vi "StageController.vi"() -> ()   [LabVIEW 2013]
panel:
  in  "Motor Port":i32=14 min=1 max=255 step=1
  out "Port\nOpen\nStatus 2":bool
  in  "moveForward":bool caption="Move Forward"
  in  "moveBackwards":bool caption="Move Backwards"
  in  "positions":string(combo) caption="Positions"
  in  "motorSpeed":dbl caption="Motor Speed (steps/s)" min=0.0 max=2000.0 format="%#.4g"
  in  "setEncodertoZero":bool caption="Set Encoder to Zero"
  in  "home":bool caption="Home"
  in  "encoderCOM":refnum<visa-resource-name>="COM13" caption="Encoder COM Port"
  in  "showTerminal":bool caption="Show Terminal"
  in  "EXIT":bool
  out "currentPos":dbl caption="Current Position (mm)" format="%.3g"
  in  "goToSelPos":bool caption="Go to Selected Position"
  in  "selPos":dbl=1.0 caption="Selected Position  (mm)" min=1.0 max=4060.0 format="%.3g"
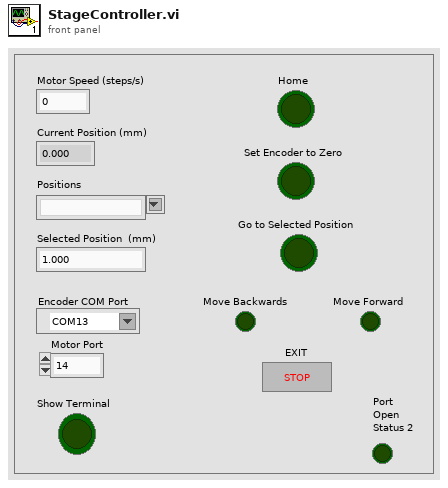
[diagram p1: front panel]
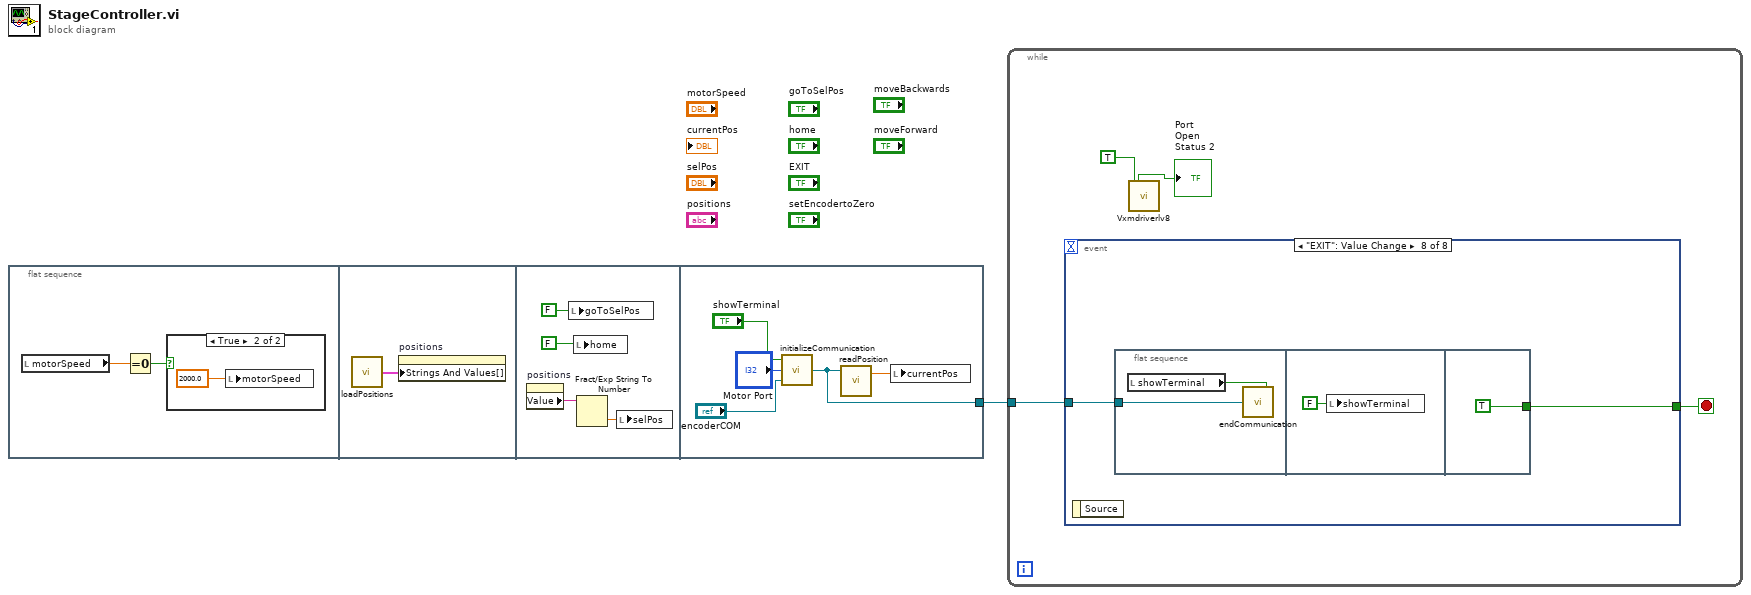
[diagram p0: block diagram]
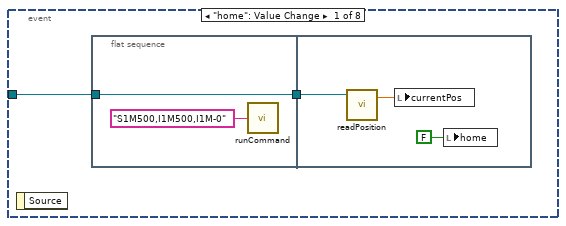
[diagram p3: hidden frame]
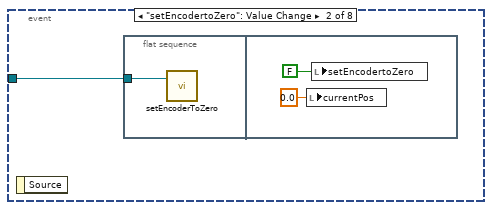
[diagram p4: hidden frame]
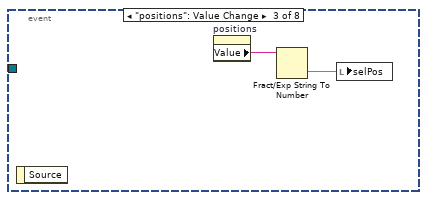
[diagram p5: hidden frame]
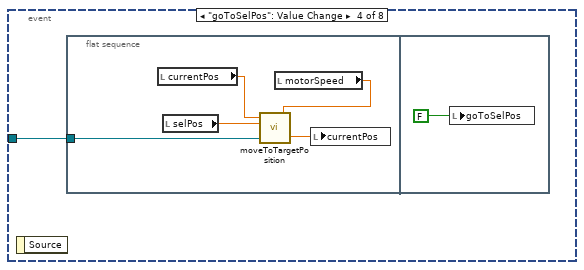
[diagram p6: hidden frame]
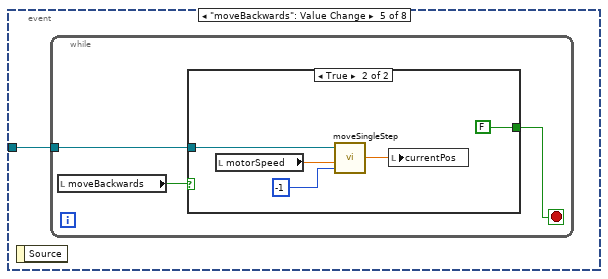
[diagram p7: hidden frame]
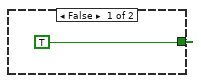
[diagram p8: hidden frame]
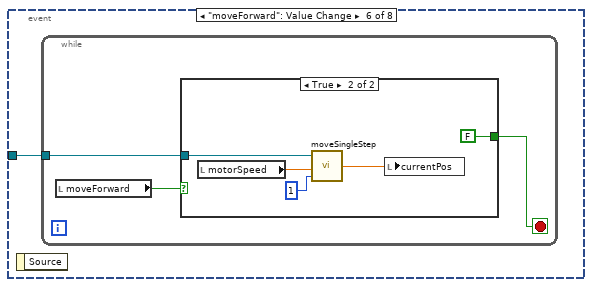
[diagram p9: hidden frame]
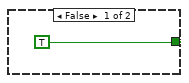
[diagram p10: hidden frame]
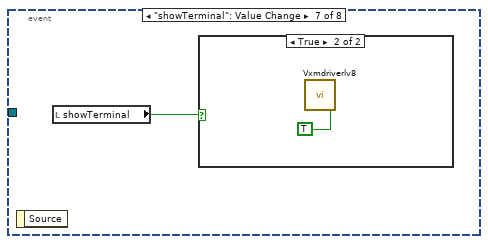
[diagram p11: hidden frame]
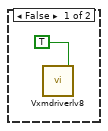
[diagram p12: hidden frame]
diagram:
  n1 = flat-sequence {
    tunnel: [w11] -> w1
    frame #0 {
      n2 = local read "motorSpeed"() -> (w2:dbl)
      n3 = Equal To 0?(x=w2) -> (x = 0?=w3:bool)
      n4 = case shown="True" w3 {
        frame False {
        }
        frame True {
          n5 = local write "motorSpeed"(2000.0 ("Motor Speed")) -> ()
        }
      }
    }
    frame #1 {
      n6 = call "loadPositions.vi"() -> ("positions"=w5:cluster{string, string}[])
      n7 = property on="positions" class="CmbBox"("Strings And Values[]"=w5) -> ()  [unwired: 2 in, 2 out]
    }
    frame #2 {
      n8 = property on="positions" class="CmbBox"() -> ("Value"=w7:string)  [unwired: 2 in, 2 out]
      n9 = local write "goToSelPos"(FALSE ("goToPos1")) -> ()
      n10 = local write "home"(FALSE ("Home")) -> ()
      n11 = Fract/Exp String To Number(string=w7) -> (number=w6:dbl)  [unwired: 3 in, 1 out]
      n12 = local write "selPos"(w6) -> ()
    }
    frame #3 {
      n13 = call "initializeCommunication.vi"("Encoder COM Port"="encoderCOM", "Port"="Motor Port", "Show Terminal"="showTerminal") -> ("Encoder VISA Resource Name (out)"=w11:refnum<visa-resource-name>)
      n14 = call "readPosition.vi"("VISA resource name"=w11) -> ("position"=w12:dbl)  [unwired: 1 in, 2 out]
      n15 = local write "currentPos"(w12) -> ()
    }
  }
  n16 = while {
    tunnel: w1 -> [w18]
    stop <- w17 stop-if-true
    n17 = event shown="[7] \"EXIT\": Value Change" {
      selector: _ -> [_ _ _ _ _ _ _ _]
      dyn-events: _ -> [_ _ _ _ _ _ _ _]
      timeout: _ -> [_ _ _ _ _ _ _ _]
      tunnel: w18 -> [w19 w26 _ w32 w39 w49 _ w63]
      tunnel: [_ _ _ _ _ _ _ w62] -> w17
      event "home": Value Change {
        n18 = event-data() -> ()  [unwired: 1 in, 1 out]
        n19 = flat-sequence {
          tunnel: [w21] -> w20
          tunnel: w19 -> [w21]
          tunnel: w20 -> [w23]
          frame #0 {
            n20 = call "runCommand.vi"("command"="S1M500,I1M500,I1M-0") -> ()  [unwired: 1 in]
          }
          frame #1 {
            n21 = call "readPosition.vi"("VISA resource name"=w23) -> ("position"=w24:dbl)  [unwired: 1 in, 2 out]
            n22 = local write "currentPos"(w24) -> ()
            n23 = local write "home"(FALSE ("Home")) -> ()
          }
        }
      }
      event "setEncodertoZero": Value Change {
        n24 = event-data() -> ()  [unwired: 1 in, 1 out]
        n25 = flat-sequence {
          tunnel: w26 -> [w27]
          frame #0 {
            n26 = call "setEncoderToZero.vi"("VISA resource name"=w27) -> ()  [unwired: 1 in, 2 out]
          }
          frame #1 {
            n27 = local write "currentPos"(0.0 ("currentPos")) -> ()
            n28 = local write "setEncodertoZero"(FALSE ("Set Encoder to Zero")) -> ()
          }
        }
      }
      event "positions": Value Change {
        n29 = event-data() -> ()  [unwired: 1 in, 1 out]
        n30 = property on="positions" class="CmbBox"() -> ("Value"=w31:string)  [unwired: 2 in, 2 out]
        n31 = Fract/Exp String To Number(string=w31) -> (number=w30:dbl)  [unwired: 3 in, 1 out]
        n32 = local write "selPos"(w30) -> ()
      }
      event "goToSelPos": Value Change {
        n33 = event-data() -> ()  [unwired: 1 in, 1 out]
        n34 = flat-sequence {
          tunnel: w32 -> [w34]
          frame #0 {
            n35 = local read "currentPos"() -> (w37:dbl)
            n36 = local read "selPos"() -> (w33:dbl)
            n37 = local read "motorSpeed"() -> (w35:dbl)
            n38 = call "moveToTargetPosition.vi"("speed"=w35, "Encoder COM Port"=w34, "targetPos"=w33, "currentPos"=w37) -> ("updatedCurrentPos"=w36:dbl)
            n39 = local write "currentPos"(w36) -> ()
          }
          frame #1 {
            n40 = local write "goToSelPos"(FALSE ("goToPos3")) -> ()
          }
        }
      }
      event "moveBackwards": Value Change {
        n41 = event-data() -> ()  [unwired: 1 in, 1 out]
        n42 = while {
          tunnel: w39 -> [w41]
          stop <- w42 stop-if-true
          n43 = local read "moveBackwards"() -> (w40:bool)
          n44 = case shown="True" w40 {
            tunnel: [TRUE FALSE] -> w42
            tunnel: w41 -> [_ w47]
            frame False {
            }
            frame True {
              n45 = local read "motorSpeed"() -> (w44:dbl)
              n46 = call "moveSingleStep.vi"("direction"=-1, "motorSpeed"=w44, "VISA resource name"=w47) -> ("position"=w45:dbl)
              n47 = local write "currentPos"(w45) -> ()
            }
          }
        }
      }
      event "moveForward": Value Change {
        n48 = event-data() -> ()  [unwired: 1 in, 1 out]
        n49 = while {
          tunnel: w49 -> [w50]
          stop <- w52 stop-if-true
          n50 = local read "moveForward"() -> (w51:bool)
          n51 = case shown="True" w51 {
            tunnel: [TRUE FALSE] -> w52
            tunnel: w50 -> [_ w57]
            frame False {
            }
            frame True {
              n52 = local read "motorSpeed"() -> (w54:dbl)
              n53 = call "moveSingleStep.vi"("direction"=1, "motorSpeed"=w54, "VISA resource name"=w57) -> ("position"=w55:dbl)
              n54 = local write "currentPos"(w55) -> ()
            }
          }
        }
      }
      event "showTerminal": Value Change {
        n55 = event-data() -> ()  [unwired: 1 in, 1 out]
        n56 = local read "showTerminal"() -> (w59:bool)
        n57 = case shown="True" w59 {
          frame False {
            n58 = call "Vxmdriverlv8.Vi"("Hide Terminal"=TRUE) -> ()  [unwired: 21 in, 6 out]
          }
          frame True {
            n59 = call "Vxmdriverlv8.Vi"("Show Terminal"=TRUE) -> ()  [unwired: 21 in, 6 out]
          }
        }
      }
      event "EXIT": Value Change {
        n60 = event-data() -> ()  [unwired: 1 in, 1 out]
        n61 = flat-sequence {
          tunnel: w63 -> [w65]
          tunnel: [TRUE] -> w62
          frame #0 {
            n62 = local read "showTerminal"() -> (w64:bool)
            n63 = call "endCommunication.vi"("Show Terminal"=w64, "Encoder COM Port"=w65) -> ()
          }
          frame #1 {
            n64 = local write "showTerminal"(FALSE ("Show Terminal")) -> ()
          }
          frame #2 {
          }
        }
      }
    }
    n65 = call "Vxmdriverlv8.Vi"("Is Port Open"=TRUE) -> ("Port\nOpen\nStatus"=→"Port\nOpen\nStatus 2":bool)  [unwired: 21 in, 5 out]
  }
